vi "GetText.vi"(8 "error in":errorcluster, 11 "channel in":refnum<class "_Channel.lvclass">) -> (0 "error out":errorcluster, 1 "additional text":string, 2 "text":string, 3 "channel out":refnum<class "_Channel.lvclass">, 4 "glyph":string)   [LabVIEW 2013, in "_Channel.lvclass"]
uses:
  _Channel.lvclass
  _Channel.lvclass/_Channel.ctl
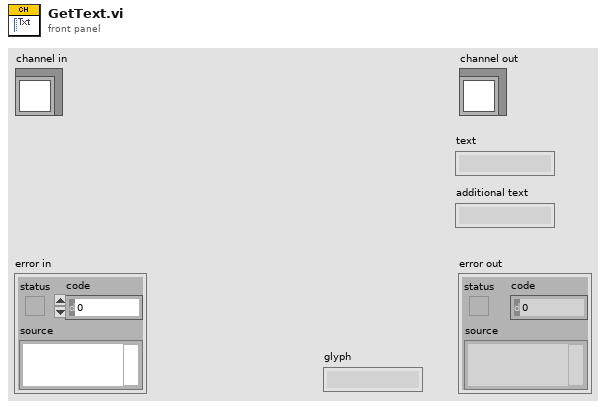
[diagram p1: front panel]
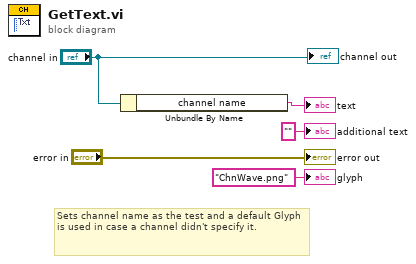
[diagram p0: block diagram]
diagram:
  # "Sets channel name as the test and a default Glyph is used in case a channel didn't specify it."
  n1 = Unbundle By Name("channel in") -> ("channel name"=→"text":string)
  "error out" <- "error in"
  "channel out" <- "channel in"
  "additional text" <- "" ("additional text")
  "glyph" <- "ChnWave.png" ("glyph")
